vi "Save Test Sequence (SubVI).vi"(7 "References":T1) -> (15 "Save Test Error":errorcluster)   [LabVIEW 2010]
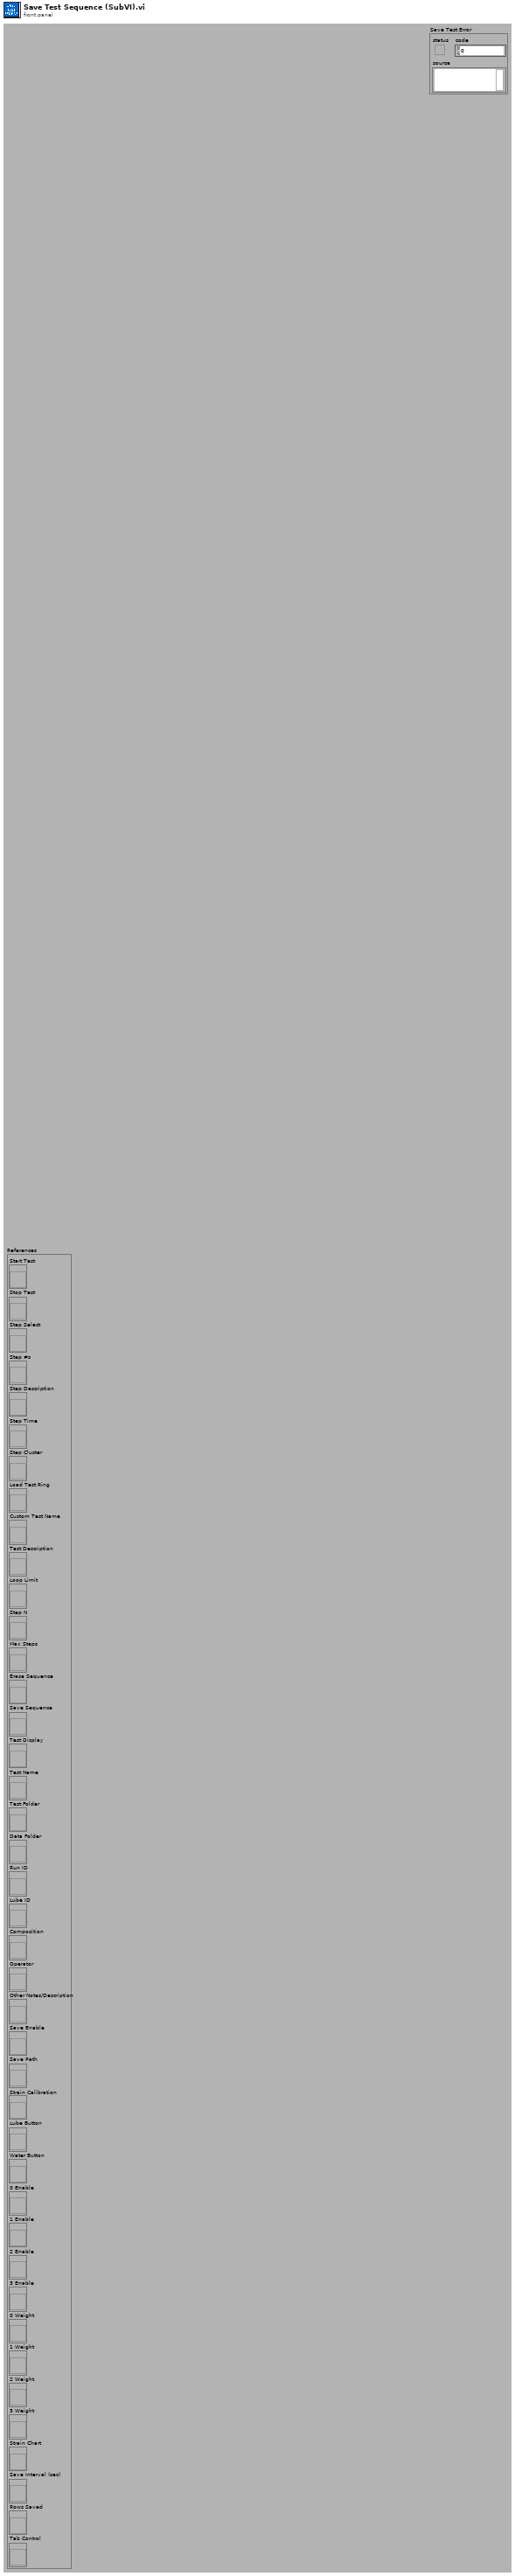
[diagram p1: front panel]
types:
  T1 = cluster{"Start Test":refnum<vi>, "Stop Test":refnum<vi>, "Step Select":refnum<vi>, "Step #s":refnum<vi>, "Step Description":refnum<vi>, "Step Time":refnum<vi>, "Step Cluster":refnum<vi>, "Load Test Ring":refnum<vi>, "Custom Test Name":refnum<vi>, "Test Description":refnum<vi>, "Loop Limit":refnum<vi>, "Step N":refnum<vi>, "Max Steps":refnum<vi>, "Erase Sequence":refnum<vi>, "Save Sequence":refnum<vi>, "Test Display":refnum<vi>, "Test Name":refnum<vi>, "Test Folder":refnum<vi>, "Data Folder":refnum<vi>, "Run ID":refnum<vi>, "Lube ID":refnum<vi>, "Composition":refnum<vi>, "Operator":refnum<vi>, "Other Notes/Description":refnum<vi>, "Save Enable":refnum<vi>, "Save Path":refnum<vi>, "Strain Calibration":refnum<vi>, "Lube Button":refnum<vi>, "Water Button":refnum<vi>, "0 Enable":refnum<vi>, "1 Enable":refnum<vi>, "2 Enable":refnum<vi>, "3 Enable":refnum<vi>, "0 Weight":refnum<vi>, "1 Weight":refnum<vi>, "2 Weight":refnum<vi>, "3 Weight":refnum<vi>, "Strain Chart":refnum<vi>, "Save Interval (sec)":refnum<vi>, "Rows Saved":refnum<vi>, "Tab Control":refnum<vi>}
  T2 = enum16{"open", "replace", "create", "open or create", "replace or create", "replace or create with confirmation"}
  T3 = cluster{"Step Time Unit":u16, "Step End Action":u16, "Relay1":bool, "Relay2":bool}[]
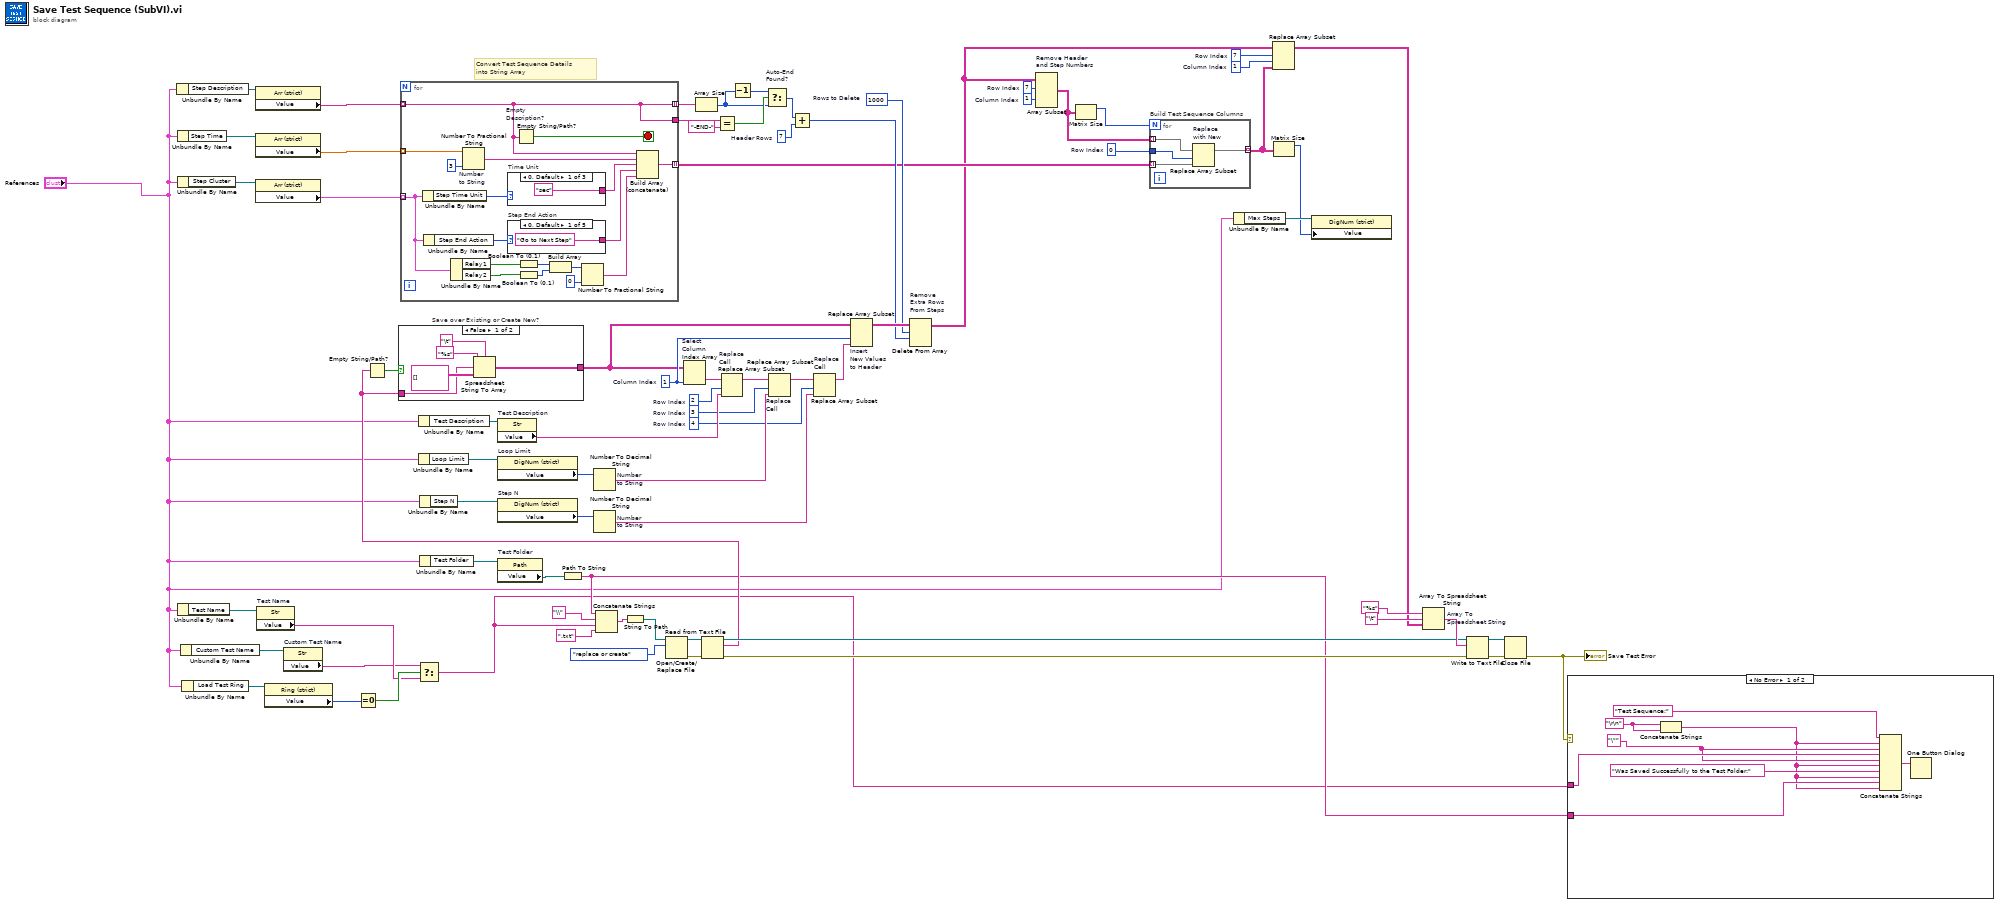
[diagram p0: block diagram]
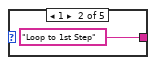
[diagram p3: hidden frame]
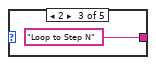
[diagram p4: hidden frame]
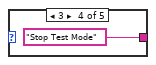
[diagram p5: hidden frame]
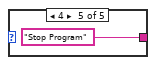
[diagram p6: hidden frame]
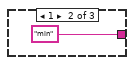
[diagram p7: hidden frame]
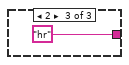
[diagram p8: hidden frame]
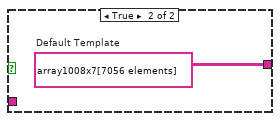
[diagram p9: hidden frame]
diagram:
  w48 = 7  # Header Rows
  w49 = 1000  # Rows to Delete
  w52 = 2  # Row Index
  w63 = 4  # Row Index
  w70 = 3  # Row Index
  w69 = 1  # Column Index
  w71 = 0  # Row Index
  w72 = 1  # Column Index
  w73 = 7  # Row Index
  w74 = 1  # Column Index
  w75 = 7  # Row Index
  # "Convert Test Sequence Details\ninto String Array"
  n1 = Unbundle By Name("References") -> ("Step Description"=w46:refnum<vi>)
  n2 = Unbundle By Name("References") -> ("Step Time"=w44:refnum<vi>)
  n3 = Unbundle By Name("References") -> ("Step Cluster"=w42:refnum<vi>)
  n4 = Unbundle By Name("References") -> ("Test Name"=w14:refnum<vi>)
  n5 = Unbundle By Name("References") -> ("Custom Test Name"=w6:refnum<vi>)
  n6 = Unbundle By Name("References") -> ("Load Test Ring"=w10:refnum<vi>)
  n7 = property class="Arr (strict)"(reference=w46) -> ("Value"=w45:string[])  [unwired: 1 in, 2 out]
  n8 = property class="Arr (strict)"(reference=w44) -> ("Value"=w43:dbl[])  [unwired: 1 in, 2 out]
  n9 = property class="Arr (strict)"(reference=w42) -> ("Value"=w41:T3)  [unwired: 1 in, 2 out]
  n10 = property on="Test Name" class="Str"(reference=w14) -> ("Value"=w7:string)  [unwired: 1 in, 2 out]
  n11 = property class="Ring (strict)"(reference=w10) -> ("Value"=w9:u16)  [unwired: 1 in, 2 out]
  n12 = property on="Custom Test Name" class="Str"(reference=w6) -> ("Value"=w5:string)  [unwired: 1 in, 2 out]
  n13 = Equal To 0?(x=w9) -> (x = 0?=w8:bool)
  n14 = for {
    tunnel: w45 -> [w78] mode=indexing
    tunnel: w43 -> [w91] mode=indexing
    tunnel: w41 -> [w90] mode=indexing
    tunnel: [w79] -> w36 mode=indexing
    tunnel: [w78] -> w40 mode=indexing
    tunnel: [w78] -> w31
    stop <- w77 stop-if-true
    n15 = Unbundle By Name(w90) -> ("Step Time Unit"=w94:u16)
    n16 = Unbundle By Name(w90) -> ("Step End Action"=w93:u16)
    n17 = Unbundle By Name(w90) -> ("Relay1"=w89:bool, "Relay2"=w88:bool)
    n18 = Number To Fractional String "Number\nto String"(number=w91, precision (6)=i16 3) -> (F-format string=w83:string)  [unwired: 2 in]
    n19 = case "Time Unit" shown="0, Default" w94 {
      tunnel: ["sec" "min" "hr"] -> w82
      frame 0, Default {
      }
      frame 1 {
      }
      frame 2 {
      }
    }
    n20 = case "Step End Action" shown="0, Default" w93 {
      tunnel: ["Go to Next Step" "Loop to 1st Step" "Loop to Step N" "Stop Test Mode" "Stop Program"] -> w81
      frame 0, Default {
      }
      frame 1 {
      }
      frame 2 {
      }
      frame 3 {
      }
      frame 4 {
      }
    }
    n21 = Empty String/Path? "Empty\nDescription?"(string/path=w78) -> (empty?=w77:bool)
    n22 = Boolean To (0,1)(Boolean=w89) -> (0, 1=w86:i16)
    n23 = Boolean To (0,1)(Boolean=w88) -> (0, 1=w87:i16)
    n24 = Build Array(w86, w87) -> (w85:i16[])
    n25 = Number To Fractional String(number=w85, precision (6)=i16 0) -> (F-format string=w80:string[])  [unwired: 2 in]
    n26 = Build Array (concatenate)(w78, w83, w82, w81, w80) -> (w79:string[])
  }
  n27 = Unbundle By Name("References") -> ("Test Description"=w39:refnum<vi>)
  n28 = Unbundle By Name("References") -> ("Loop Limit"=w38:refnum<vi>)
  n29 = Select(t=w5, s=w8, f=w7) -> (s? t:f=w2:string)
  n30 = Unbundle By Name("References") -> ("Step N"=w37:refnum<vi>)
  n31 = Unbundle By Name("References") -> ("Test Folder"=w22:refnum<vi>)
  n32 = property on="Test Description" class="Str"(reference=w39) -> ("Value"=w76:string)  [unwired: 1 in, 2 out]
  n33 = property on="Loop Limit" class="DigNum (strict)"(reference=w38) -> ("Value"=w68:i32)  [unwired: 1 in, 2 out]
  n34 = property on="Step N" class="DigNum (strict)"(reference=w37) -> ("Value"=w65:i32)  [unwired: 1 in, 2 out]
  n35 = property on="Test Folder" class="Path"(reference=w22) -> ("Value"=w21:path)  [unwired: 1 in, 2 out]
  n36 = Path To String(path=w21) -> (string=w3:string)
  n37 = Number To Decimal String "Number\nto String"(number=w68) -> (decimal integer string=w67:string)  [unwired: 1 in]
  n38 = Number To Decimal String "Number\nto String"(number=w65) -> (decimal integer string=w64:string)  [unwired: 1 in]
  n39 = Concatenate Strings(w3, "\\" ("string"), w2, ".txt" ("string")) -> (w16:string)
  n40 = String To Path(string=w16) -> (path=w20:path)
  n41 = Open/Create/Replace File(file path (use dialog)=w20, operation (0:open)=T2."replace or create") -> (refnum out=w19:refnum<file>, error out=w17:errorcluster)  [unwired: 4 in, 1 out]
  n42 = Array Size(array=w40) -> (size(s)=w28:i32)
  n43 = Read from Text File(file (use dialog)=w19, error in=w17) -> (refnum out=w58:refnum<file>, text=w57:string, error out=w55:errorcluster)  [unwired: 3 out]
  n44 = Empty String/Path?(string/path=w57) -> (empty?=w23:bool)
  n45 = case "Save over Existing or Create New?" shown="False" w23 {
    tunnel: w57 -> [w104 _]
    tunnel: [w103 w108] -> w56
    frame False {
      n46 = Spreadsheet String To Array(delimiter (Tab)="\t" ("delimiter (\\t)"), format string="%s" ("format (%s)"), spreadsheet string=w104, array type (2D Dbl)=string[][] [] ("appended array")) -> (array=w103:string[][])
    }
    frame True {
      w108 = string[][] array1008x7[7056 elements]  # Default Template
    }
  }
  n47 = Index Array "Select\nColumn"(array=w56, index (col)=w69) -> (element=w54:string[])  [unwired: 1 in]
  n48 = Equal?(x=w31, y="-END-") -> (x = y?=w30:bool)
  n49 = Replace Array Subset "Replace\nCell"(array=w54, new element=w76, index=w52) -> (w53:string[])
  n50 = Decrement(x=w28) -> (x-1=w29:i32)
  n51 = Select "Auto-End\nFound?"(t=w29, s=w30, f=w28) -> (s? t:f=w27:i32)
  n52 = Replace Array Subset "Replace\nCell"(array=w53, new element=w67, index=w70) -> (w66:string[])
  n53 = Add(x=w27, y=w48) -> (x+y=w47:i32)
  n54 = Replace Array Subset "Replace\nCell"(array=w66, new element=w64, index=w63) -> (w62:string[])
  n55 = Replace Array Subset "Insert\nNew Values\nto Header"(array=w56, new element=w62, index (col)=w69) -> (w50:string[][])  [unwired: 1 in]
  n56 = Delete From Array "Remove\nExtra Rows\nFrom Steps"(array=w50, length=w49, index (row)=w47) -> (array with subset deleted=w35:string[][])  [unwired: 1 in, 1 out]
  n57 = Array Subset "Remove Header\nand Step Numbers"(array=w35, index (row)=w75, index (col)=w74) -> (w34:string[][])  [unwired: 2 in]
  n58 = Matrix Size(0:w34) -> (1:w33:i32)  [unwired: 1 out]
  n59 = for "Build Test Sequence Columns" {
    N: w33 -> [_]
    tunnel: w34 -> [w109] mode=indexing
    tunnel: w36 -> [w112] mode=indexing
    tunnel: [w110] -> w26 mode=indexing
    tunnel: w71 -> [w111]
    n60 = Replace Array Subset "Replace\nwith New"(array=w109, new element=w112, index=w111) -> (w110:string[])
  }
  n61 = Unbundle By Name("References") -> ("Max Steps"=w12:refnum<vi>)
  n62 = Replace Array Subset "Replace Array Subset"(array=w35, new element=w26, index (row)=w73, index (col)=w72) -> (w51:string[][])
  n63 = Matrix Size(0:w26) -> (1:w11:i32)  [unwired: 1 out]
  n64 = property class="DigNum (strict)"(reference=w12, "Value"=w11) -> ()  [unwired: 1 in, 2 out]
  n65 = Array To Spreadsheet String "Array To \nSpreadsheet String"(delimiter (Tab)="\t" ("delimiter (\\t)"), array=w51, 3:"%s" ("format (%s)")) -> (spreadsheet string=w59:string)
  n66 = Write to Text File(file (use dialog)=w58, text=w59, error in=w55) -> (refnum out=w25:refnum<file>, error out=w24:errorcluster)  [unwired: 1 in, 1 out]
  n67 = Close File(refnum=w25, error in=w24) -> (error out=w4:errorcluster)  [unwired: 1 out]
  "Save Test Error" <- w4
  n68 = case shown="No Error" w4 {
    tunnel: w3 -> [w114 _]
    tunnel: w2 -> [w117 _]
    frame No Error {
      w119 = "\r\n"
      w116 = "\""
      n69 = Concatenate Strings(w119, w119) -> (w113:string)
      n70 = Concatenate Strings("Test Sequence:", w113, w116, w117, w116, w113, "Was Saved Successfully to the Test Folder:", w113, w114, w113) -> (w120:string)
      n71 = One Button Dialog(message=w120) -> ()  [unwired: 1 in, 1 out]
    }
    frame Error {
    }
  }
